vi "xxPololuCommand.vi"(4 "Channel Name":string="Aalborg", 6 "Port Name":string="mfc1", 8 "Numeric Value":i32, 9 "PololuCommand":T4="FullScaleRatingSLPM", 10 "Address":u8) -> (0 "String Reply":string="!11,100.0000\r\n")   [LabVIEW 2018]
uses:
  PololuActions.ctl
  PololuCommandDescriptor.ctl
  TicCommandType.ctl
  PololuCommand.ctl
panel:
  out "Audit":T1[](array[typedef])
  out "Case":T1
  out "SendString":string="!11,100.0000\r\n"
  out "In Range?":bool
  out "CommandDescriptorOutput":T2={"PololuCommand"="FullScaleRatingSLPM", "Mnemonic"="", "CommandType"=enum."Command", "Min"=2147483647, "Max"=0}
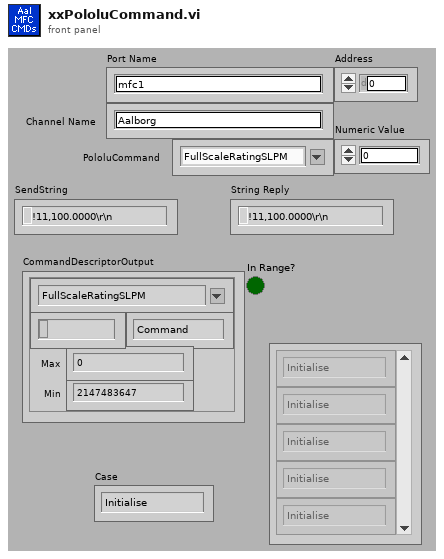
[diagram p1: front panel]
types:
  T1 = typedef "PololuActions.ctl" = enum16{"Initialise", "GetCommand", "CheckLimits", "Encode", "Send", "Decode", "Done"}
  T2 = typedef "PololuCommandDescriptor.ctl" = cluster{"PololuCommand":string, "Mnemonic":string, "CommandType":T3, "Min":i32, "Max":i32}
  T3 = typedef "TicCommandType.ctl" = enum16{"Command", "7-bitWrite", "32-bitWrite", "BlockRead"}
  T4 = typedef "PololuCommand.ctl" = string
  T5 = enum16{"Quick", "7-bitWrite", "32-bitWrite", "BlockRead"}
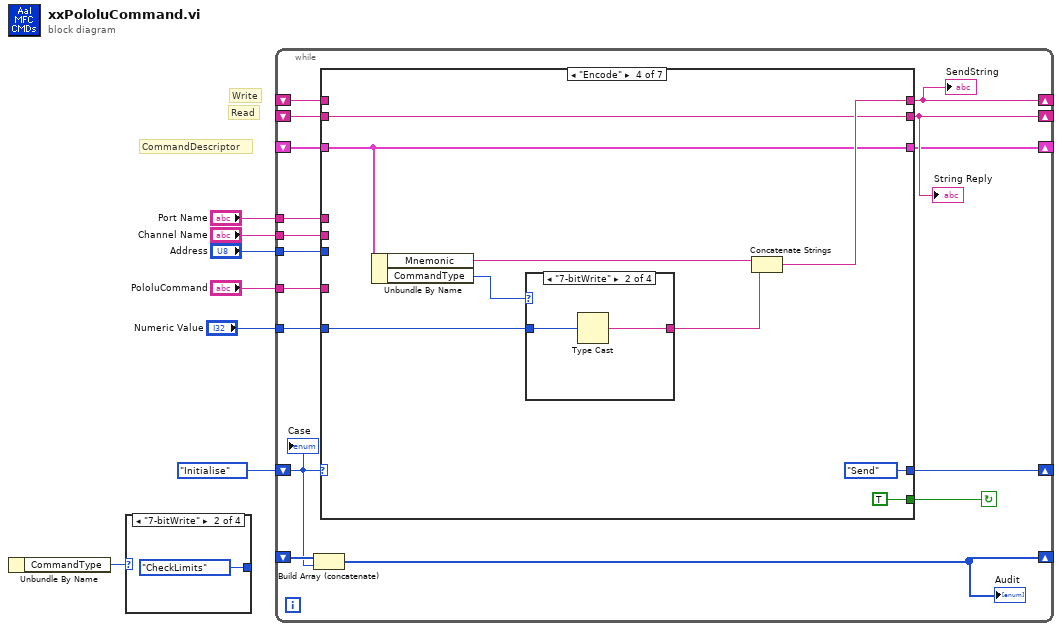
[diagram p0: block diagram]
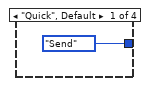
[diagram p2: hidden frame]
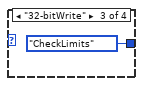
[diagram p3: hidden frame]
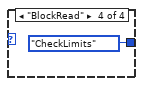
[diagram p4: hidden frame]
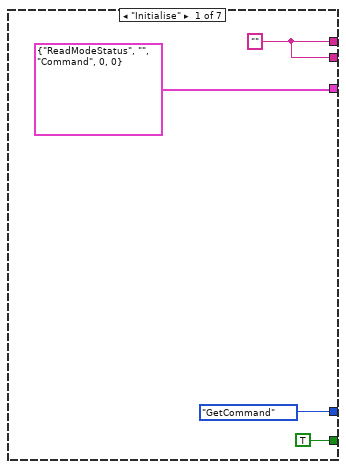
[diagram p5: hidden frame]
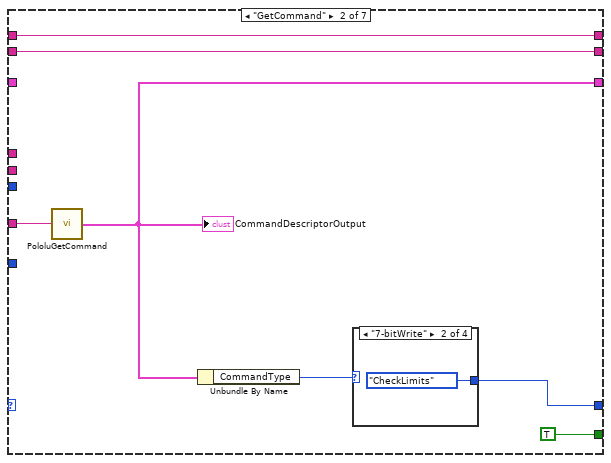
[diagram p6: hidden frame]
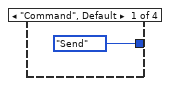
[diagram p7: hidden frame]
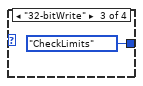
[diagram p8: hidden frame]
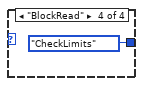
[diagram p9: hidden frame]
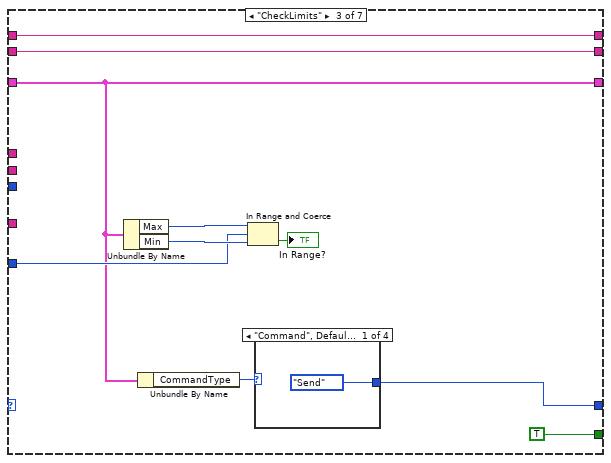
[diagram p10: hidden frame]
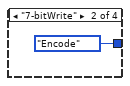
[diagram p11: hidden frame]
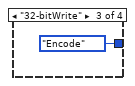
[diagram p12: hidden frame]
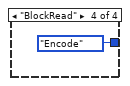
[diagram p13: hidden frame]
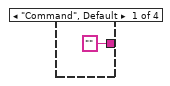
[diagram p14: hidden frame]
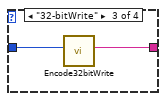
[diagram p15: hidden frame]
diagram:
  # "CommandDescriptor"
  # "Read"
  # "Write"
  n1 = Unbundle By Name() -> ("CommandType"=w1:T5)  [unwired: 1 in]
  n2 = case shown="\"7-bitWrite\"" w1 {
    tunnel: [PololuActions."Send" ("Combo Box") PololuActions."CheckLimits" ("Combo Box") PololuActions."CheckLimits" ("Combo Box") PololuActions."CheckLimits" ("Combo Box")] -> _
    frame "Quick", Default {
    }
    frame "7-bitWrite" {
    }
    frame "32-bitWrite" {
    }
    frame "BlockRead" {
    }
  }
  n3 = while {
    shift-right: [w19] -> _
    shift-left: PololuActions."Initialise" ("Combo Box") -> [w13]
    tunnel: "Address" -> [w27]
    tunnel: "PololuCommand" -> [w26]
    shift-right: [w14] -> _
    shift-left: _ -> [w25]
    tunnel: "Port Name" -> [w24]
    tunnel: "Channel Name" -> [w23]
    shift-right: [w18] -> _
    shift-left: _ -> [w22]
    shift-right: [w12] -> _
    shift-left: _ -> [w20]
    shift-right: [w17] -> _
    shift-left: _ -> [w16]
    tunnel: "Numeric Value" -> [w15]
    stop <- w21 continue-if-true
    n4 = Build Array (concatenate)(w20, w13) -> (w12:T1[])
    "Audit" <- w12
    n5 = case shown="\"Encode\"" w13 {
      tunnel: [PololuActions."GetCommand" ("Combo Box") w32 w43 PololuActions."Send" ("Combo Box") _ _ _] -> w19
      tunnel: w27 -> [_ _ _ _ _ _ _]
      tunnel: w26 -> [_ w35 _ _ _ _ _]
      tunnel: [w31 w37 w50 w62 _ _ _] -> w14
      tunnel: w25 -> [_ w37 w50 _ _ _ _]
      tunnel: w24 -> [_ _ _ _ _ _ _]
      tunnel: w23 -> [_ _ _ _ _ _ _]
      tunnel: [w31 w36 w52 w61 _ _ _] -> w18
      tunnel: w22 -> [_ w36 w52 w61 _ _ _]
      tunnel: [TRUE ("Continue") TRUE ("Continue") TRUE TRUE ("Continue") _ _ _] -> w21
      tunnel: [T2 {"PololuCommand"="ReadModeStatus", "Mnemonic"="", "CommandType"=enum."Command", "Min"=0, "Max"=0} ("CommandDescriptor") w34 w44 w60 _ _ _] -> w17
      tunnel: w16 -> [_ _ w44 w60 _ _ _]
      tunnel: w15 -> [_ _ w47 w65 _ _ _]
      frame "Initialise" {
        w31 = ""
      }
      frame "GetCommand" {
        n6 = call "PololuGetCommand.vi"("PololuCommand"=w35) -> ("CommandDescriptor"=w34:T2)  [unwired: 3 in, 1 out]
        "CommandDescriptorOutput" <- w34
        n7 = Unbundle By Name(w34) -> ("CommandType"=w33:T3)
        n8 = case shown="\"7-bitWrite\"" w33 {
          tunnel: [PololuActions."Send" ("Combo Box") PololuActions."CheckLimits" ("Combo Box") PololuActions."CheckLimits" ("Combo Box") PololuActions."CheckLimits" ("Combo Box")] -> w32
          frame "Command", Default {
          }
          frame "7-bitWrite" {
          }
          frame "32-bitWrite" {
          }
          frame "BlockRead" {
          }
        }
      }
      frame "CheckLimits" {
        n9 = Unbundle By Name(w44) -> ("Max"=w49:i32, "Min"=w48:i32)
        n10 = Unbundle By Name(w44) -> ("CommandType"=w45:T3)
        n11 = In Range and Coerce(upper limit=w49, x=w47, lower limit=w48) -> (In Range?=→"In Range?":bool)  [unwired: 1 out]
        n12 = case shown="\"Command\", Default" w45 {
          tunnel: [PololuActions."Send" ("Combo Box") PololuActions."Encode" ("Combo Box") PololuActions."Encode" ("Combo Box") PololuActions."Encode" ("Combo Box")] -> w43
          frame "Command", Default {
          }
          frame "7-bitWrite" {
          }
          frame "32-bitWrite" {
          }
          frame "BlockRead" {
          }
        }
      }
      frame "Encode" {
        n13 = Unbundle By Name(w60) -> ("Mnemonic"=w64:string, "CommandType"=w57:T3)
        n14 = case shown="\"7-bitWrite\"" w57 {
          tunnel: w65 -> [_ w68 w70 _]
          tunnel: ["" ("PololuString") w67 w69 _] -> w63
          frame "Command", Default {
          }
          frame "7-bitWrite" {
            n15 = Type Cast(x=w68) -> (*(type *) &x=w67:string)  [unwired: 1 in]
          }
          frame "32-bitWrite" {
            n16 = call "Encode32bitWrite.vi"("Numeric"=w70) -> ("PololuString"=w69:string)  [unwired: 10 in]
          }
          frame "BlockRead" {
          }
        }
        n17 = Concatenate Strings(w64, w63) -> (w62:string)
      }
      frame "Send" {
      }
      frame "Decode" {
      }
      frame "Done" {
      }
    }
    "String Reply" <- w18
    "SendString" <- w14
    "Case" <- w13
  }
